vi "Initialize.vi"(8 "error in (no error)":errorcluster, 11 "VISA resource name":refnum<visa-resource-name>) -> (0 "error out":errorcluster, 3 "VISA resource name out":refnum<visa-resource-name>)   [LabVIEW 2013, in "Ocean Optics 2000 4000.lvlib"]
doc: "Establishes communication with the instrument and optionally performs an instrument identification query and/or an instrument reset. It also places the instrument in a default state needed for other instrument driver operations. Therefore, call this VI before calling other instrument driver VIs for this instrument. Generally, you need to call the Initialize VI only once at the beginning of an application."
uses:
  <instrlib>/Ocean Optics 2000 4000/Ocean Optics 2000 4000.lvlib
panel:
  in  "General Settings:Model Code":u16=4098
  # "(c) 2009 -2013 National Instruments.  ALL RIGHTS RESERVED."
  # "Before using this driver:\n    * Go to Program Files >>National Instruments >>LabVIEW >> \n       instr.lib>> Ocean Optics 2000 4000>>VISA_USB\n    * Select the folder for the model of instrument you are using.\n    * For Windows Vista, use the INF file with _vista in the file name\n      (eg.Ocean Optics USB4000_vista.inf). For XP, use the other INF file.\n    * To install, right click and select Install.\n    * NI MAX should be able to detect this instrument after installing the \n      INF file."
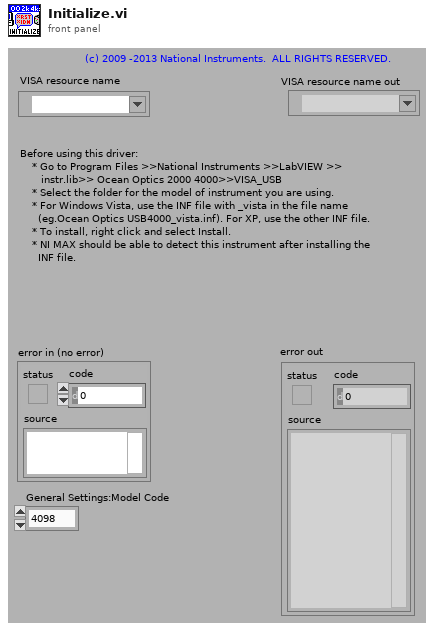
[diagram p1: front panel]
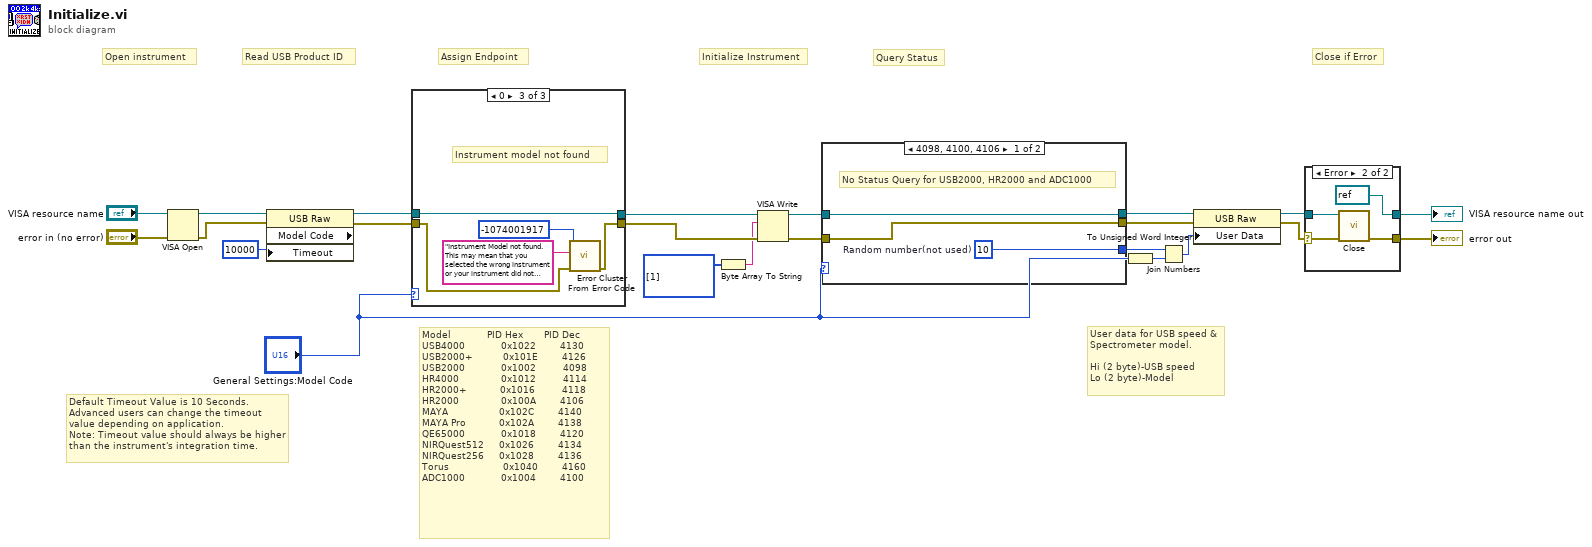
[diagram p0: block diagram]
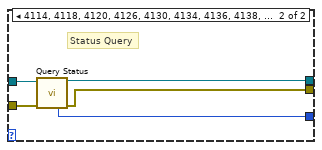
[diagram p2: hidden frame]
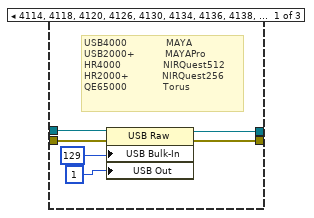
[diagram p3: hidden frame]
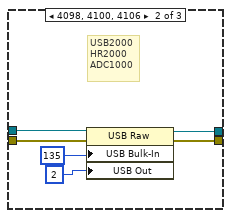
[diagram p4: hidden frame]
diagram:
  # "Default Timeout Value is 10 Seconds. Advanced users can change the timeout value depending on application.\nNote: Timeout value should always be higher than the instrument's integration time."
  # "Model            PID Hex       PID Dec \nUSB4000            0x1022        4130 \nUSB2000+          0x101E        4126 \nUSB2000            0x1002         4098\nHR4000              0x1012         4114\nHR2000+           0x1016         4118\nHR2000              0x100A        4106\nMAYA                 0x102C        4140\nMAYA Pro           0x102A        4138\nQE65000            0x1018        4120\nNIRQuest512     0x1026        4134\nNIRQuest256     0x1028        4136\nTorus                  0x1040        4160\nADC1000            0x1004        4100"
  # "Read USB Product ID"
  # "Assign Endpoint"
  # "User data for USB speed & Spectrometer model. \n\nHi (2 byte)-USB speed\nLo (2 byte)-Model"
  # "Initialize Instrument"
  # "Query Status"
  # "Close if Error"
  # "Open instrument"
  n1 = VISA Open(error in (no error)="error in (no error)", VISA resource name="VISA resource name") -> (VISA resource name=w9:refnum<visa-resource-name>, error out=w8:errorcluster)  [unwired: 3 out]
  n2 = property class="USB Raw" props=["Model Code", "Timeout"](reference=w9, error in=w8, "Timeout"=u32 10000 ("General Settings:Timeout Value")) -> (reference out=w7:refnum<visa-resource-name>, error out=w6:errorcluster)  [unwired: 1 out]
  n3 = case shown="0" "General Settings:Model Code" {
    tunnel: [w29 w31 w40] -> w20
    tunnel: [w28 w30 w39] -> w19
    tunnel: w7 -> [w27 w33 w40]
    tunnel: w6 -> [w26 w32 w36]
    frame 4114, 4118, 4120, 4126, 4130, 4134, 4136, 4138, 4140, 4160, Default {
      # "USB4000             MAYA\nUSB2000+          MAYAPro     \nHR4000              NIRQuest512\nHR2000+           NIRQuest256   \nQE65000            Torus"
      n4 = property class="USB Raw"(reference=w27, error in=w26, "USB Bulk-In"=i16 129 ("USB Settings:Bulk-In Pipe"), "USB Out"=i16 1 ("USB Settings:Bulk-In Pipe")) -> (reference out=w29:refnum<visa-resource-name>, error out=w28:errorcluster)
    }
    frame 4098, 4100, 4106 {
      # "USB2000\nHR2000\nADC1000"
      n5 = property class="USB Raw"(reference=w33, error in=w32, "USB Bulk-In"=i16 135 ("USB Settings:Bulk-In Pipe"), "USB Out"=i16 2 ("USB Settings:Bulk-In Pipe")) -> (reference out=w31:refnum<visa-resource-name>, error out=w30:errorcluster)
    }
    frame 0 {
      # "Instrument model not found"
      n6 = call <vilib>:"Error Cluster From Error Code.vi"("error in (no error)"=w36, "error message (\"\")"="Instrument Model not found.This may mean that you selected the wrong instrument or your instrument did not respond.  You may also be using a model that is not officially supported by this driver. " ("error message (\"\")"), "error code (0)"=-1074001917) -> ("error out"=w39:errorcluster)  [unwired: 6 in]
    }
  }
  n7 = Byte Array To String(unsigned byte array=u8[] [1] ("write buffer (empty)")) -> (string=w17:string)
  n8 = VISA Write(VISA resource name=w20, write buffer=w17, error in (no error)=w19) -> (VISA resource name out=w15:refnum<visa-resource-name>, error out=w14:errorcluster)  [unwired: 1 out]
  n9 = case shown="4098, 4100, 4106" "General Settings:Model Code" {
    tunnel: w15 -> [w43 w48]
    tunnel: w14 -> [w42 w47]
    tunnel: [w43 w46] -> w13
    tunnel: [w42 w45] -> w12
    tunnel: [w41 w44] -> w5
    frame 4098, 4100, 4106 {
      w41 = u16 10  # Random number(not used)
      # "No Status Query for USB2000, HR2000 and ADC1000"
    }
    frame 4114, 4118, 4120, 4126, 4130, 4134, 4136, 4138, 4140, 4160, Default {
      # "Status Query"
      n10 = call <instrlib>:"Query Status.vi"("VISA resource name"=w48, "error in (no error)"=w47) -> ("VISA resource name out"=w46:refnum<visa-resource-name>, "USB Speed"=w44:u16, "error out"=w45:errorcluster)  [unwired: 6 in, 5 out]
    }
  }
  n11 = To Unsigned Word Integer(number="General Settings:Model Code") -> (unsigned 16bit integer=w4:u16)
  n12 = Join Numbers(hi=w5, lo=w4) -> ((hi.lo)=w3:u32)
  n13 = property class="USB Raw"(reference=w13, error in=w12, "User Data"=w3) -> (reference out=w11:refnum<visa-resource-name>, error out=w10:errorcluster)
  n14 = case shown="Error" w10 {
    selector: w10 -> [w50 w53]
    tunnel: [w49 refnum<visa-resource-name> refnum ("VISA resource name out")] -> w23
    tunnel: [w50 w54] -> w22
    tunnel: w11 -> [w49 w51]
    frame No Error {
    }
    frame Error {
      n15 = call <instrlib>:"Close.vi"("error in (no error)"=w53, "VISA resource name"=w51) -> ("error out"=w54:errorcluster)  [unwired: 9 in]
    }
  }
  "VISA resource name out" <- w23
  "error out" <- w22
